vi "computeIncrementedString.vi"(10 "Input String":string, 11 "StringIncrement":refnum<class "StringIncrement.Alphabetical.lvclass">) -> (2 "Incremented String":string, 3 "StringIncrement out":refnum<class "StringIncrement.Alphabetical.lvclass">)   [LabVIEW 2014, in "StringIncrement.Alphabetical.lvclass"]
uses:
  StringIncrement.Alphabetical.lvclass
  NameIncrementAlgorithm/StringIncrement.lvclass
panel:
  out "Array":u8[](array[numeric])
  in  "Append Numeric":u32
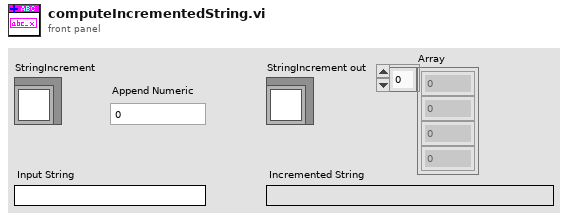
[diagram p1: front panel]
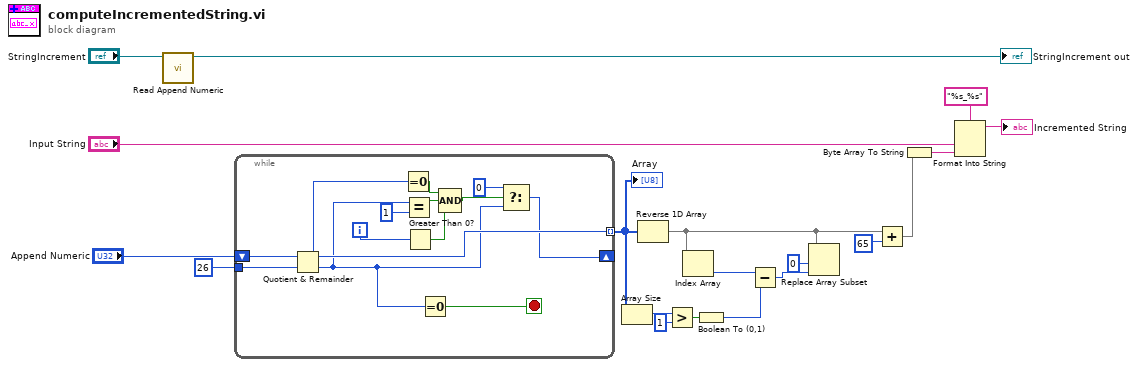
[diagram p0: block diagram]
diagram:
  n1 = call "Read Append Numeric.vi"("StringIncrement"="StringIncrement") -> ("StringIncrement out"=→"StringIncrement out":refnum<class "StringIncrement.Alphabetical.lvclass">)  [unwired: 9 in, 1 out]
  n2 = while {
    shift-right: [w21] -> _
    shift-left: "Append Numeric" -> [w30]
    tunnel: [w25] -> w3 mode=indexing
    tunnel: u32 26 ("y") -> [w31]
    i -> [w20]
    stop <- w32 stop-if-true
    n3 = Quotient & Remainder(x=w30, y=w31) -> (x-y*floor(x/y)=w25:u32, floor(x/y)=w22:u32)
    n4 = Equal To 0?(x=w25) -> (x = 0?=w28:bool)
    n5 = Equal?(x=w22, y=u32 1) -> (x = y?=w29:bool)
    n6 = Greater Than 0?(x=w20) -> (x > 0?=w23:bool)
    n7 = Equal To 0?(x=w22) -> (x = 0?=w32:bool)
    n8 = Compound Arithmetic op=AND(w28, w29, w23) -> (w27:bool)
    n9 = Select(t=u32 0, s=w27, f=w22) -> (s? t:f=w21:u32)
  }
  "Array" <- w3
  n10 = Array Size(array=w3) -> (size(s)=w7:i32)
  n11 = Reverse 1D Array(array=w3) -> (reversed array=w1:u32[])
  n12 = Greater?(x=w7, y=1) -> (0:w5:bool)
  n13 = Index Array(array=w1) -> (element=w9:u32)  [unwired: 1 in]
  n14 = Boolean To (0,1)(Boolean=w5) -> (0, 1=w4:i16)
  n15 = Subtract(x=w9, y=w4) -> (x-y=w8:u32)
  n16 = Replace Array Subset(array=w1, new element=w8, index=0) -> ()  [unwired: 1 out]
  n17 = Add(x=w1, y=u8 65) -> (x+y=w12:u32[])
  n18 = Byte Array To String(unsigned byte array=w12) -> (string=w14:string)
  n19 = Format Into String(format string="%s_%s", "Input String", w14) -> (resulting string=→"Incremented String":string)  [unwired: 2 in, 1 out]
